vi "Launcher - Main View.vi"() -> ()   [LabVIEW 2018]
uses:
  <vilib>/Utility/miscctls.llb/LVPointTypeDef.ctl
  Workers/Main View/Main View.lvclass
  D:/Program Files (x86)/National Instruments/LabVIEW 2018/vi.lib/addons/_Workers/Library/Classes/Worker/Worker.lvclass
  Workers/Aging View/Aging View.lvclass
  Workers/Query Data/Query Data.lvclass
  Workers/Save Data/Save Data.lvclass
  Workers/Acquire Data/Acquire Data.lvclass
  Workers/About View/About View.lvclass
  Workers/Settings View/Settings View.lvclass
  <vilib>/addons/_Workers/Library/Classes/Message/Enqueue Message to Self v2.vi
  <vilib>/addons/_Workers/Library/Classes/Message/Message.lvclass
  <vilib>/addons/_Workers/Debugger/Debug Client/Debug Client.lvlib
  D:/Program Files (x86)/National Instruments/LabVIEW 2018/vi.lib/addons/_Workers/Library/Classes/Workers Object/Workers Object.lvclass
panel:
  out "About View":picture caption="[About]"
  out "Query View":picture caption="[Query]"
  out "Settings View":picture caption="[Settings]"
  out "Aging View":picture caption="[Aging]"
  out "error out":errorcluster
  # "Workers Demo - Aging Test"
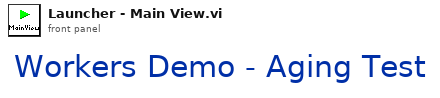
[diagram p1: front panel]
types:
  T1 = enum32{"Invalid", "Standard", "Closed", "Hidden", "Minimized", "Maximized"}
  T2 = typedef "LVPointTypeDef.ctl" = cluster{"Horizontal":i16, "Vertical":i16}
  T3 = typedef "Workers.lvlib/Case Label.ctl" = string
  T4 = typedef "imagedata.ctl" = cluster{"image type":i32, "image depth":i32, "image":u8[], "mask":u8[], "colors":u32[], "Rectangle":cluster{"left":i16, "top":i16, "right":i16, "bottom":i16}}
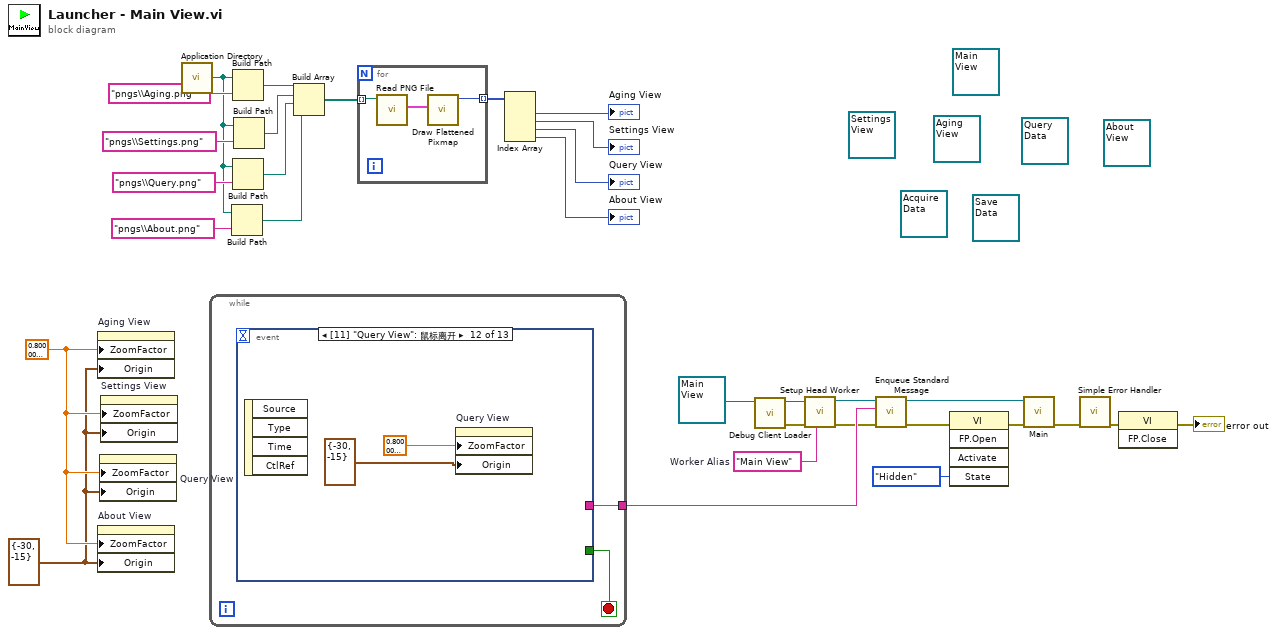
[diagram p0: block diagram]
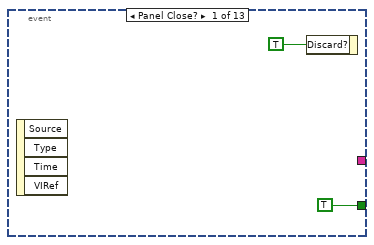
[diagram p2: hidden frame]
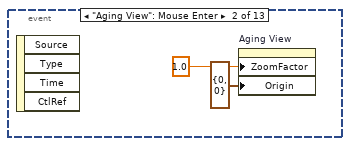
[diagram p3: hidden frame]
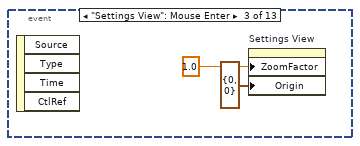
[diagram p4: hidden frame]
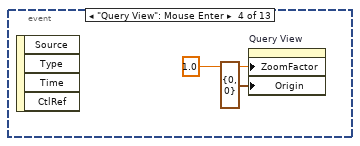
[diagram p5: hidden frame]
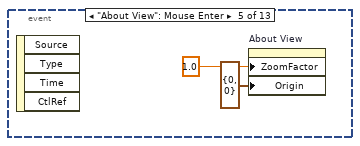
[diagram p6: hidden frame]
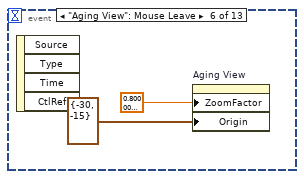
[diagram p7: hidden frame]
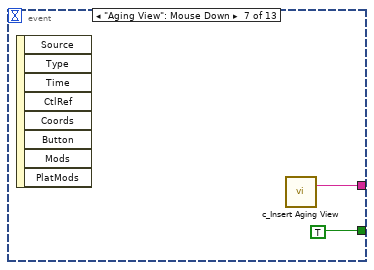
[diagram p8: hidden frame]
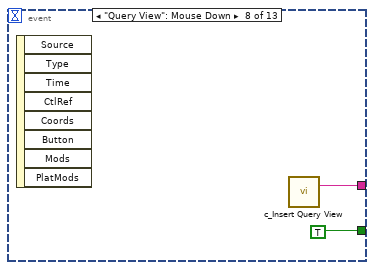
[diagram p9: hidden frame]
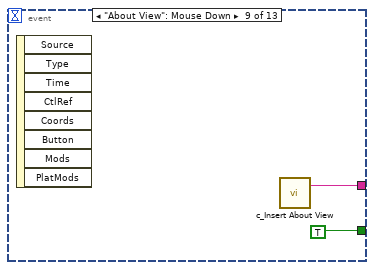
[diagram p10: hidden frame]
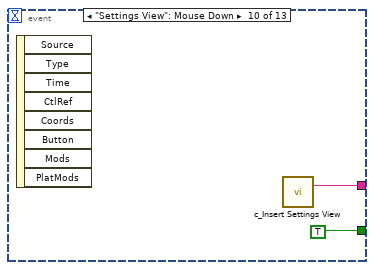
[diagram p11: hidden frame]
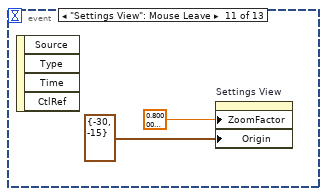
[diagram p12: hidden frame]
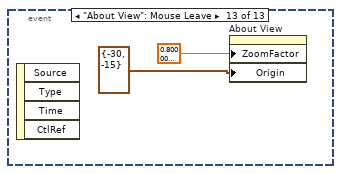
[diagram p13: hidden frame]
diagram:
  (unwired) refnum<class "Settings View.lvclass"> refnum ("Settings View.lvclass")
  (unwired) refnum<class "About View.lvclass"> refnum ("About View.lvclass")
  (unwired) refnum<class "Acquire Data.lvclass"> refnum ("Acquire Data.lvclass")
  (unwired) refnum<class "Save Data.lvclass"> refnum ("Save Data.lvclass")
  (unwired) refnum<class "Query Data.lvclass"> refnum ("Query Data.lvclass")
  (unwired) refnum<class "Main View.lvclass"> refnum ("Main View.lvclass")
  (unwired) refnum<class "Aging View.lvclass"> refnum ("Aging View.lvclass")
  w13 = "Main View"  # Worker Alias
  w15 = T2 {"Horizontal"=-30, "Vertical"=-15} ("Origin")
  w21 = sgl 0.8 ("Zoom Factor")
  n1 = property on="Aging View" class="Pict"("ZoomFactor"=w21, "Origin"=w15) -> ()  [unwired: 2 in, 2 out]
  n2 = property on="About View" class="Pict"("ZoomFactor"=w21, "Origin"=w15) -> ()  [unwired: 2 in, 2 out]
  n3 = property on="Query View" class="Pict"("ZoomFactor"=w21, "Origin"=w15) -> ()  [unwired: 2 in, 2 out]
  n4 = property on="Settings View" class="Pict"("ZoomFactor"=w21, "Origin"=w15) -> ()  [unwired: 2 in, 2 out]
  n5 = call <vilib>:"Application Directory.vi"() -> ("Application Directory"=w27:path)
  n6 = while {
    tunnel: [w32] -> w6
    stop <- w33 stop-if-true
    n7 = event shown="[11] \"Query View\": 鼠标离开" {
      selector: _ -> [_ _ _ _ _ _ _ _ _ _ _ _ _]
      dyn-events: _ -> [_ _ _ _ _ _ _ _ _ _ _ _ _]
      timeout: _ -> [_ _ _ _ _ _ _ _ _ _ _ _ _]
      tunnel: [TRUE _ _ _ _ _ TRUE TRUE TRUE TRUE _ _ _] -> w33
      tunnel: [_ _ _ _ _ _ w46 w48 w50 w52 _ _ _] -> w32
      event Panel Close? {
        n8 = event-data() -> ()  [unwired: 1 in, 4 out]
        n9 = event-data("Discard?"=TRUE) -> ()  [unwired: 1 in, 1 out]
      }
      event "Aging View": Mouse Enter {
        n10 = event-data() -> ()  [unwired: 1 in, 4 out]
        n11 = property on="Aging View" class="Pict"("ZoomFactor"=sgl 1.0 ("Zoom Factor"), "Origin"=T2 {"Horizontal"=0, "Vertical"=0}) -> ()  [unwired: 2 in, 2 out]
      }
      event "Settings View": Mouse Enter {
        n12 = event-data() -> ()  [unwired: 1 in, 4 out]
        n13 = property on="Settings View" class="Pict"("ZoomFactor"=sgl 1.0 ("Zoom Factor"), "Origin"=T2 {"Horizontal"=0, "Vertical"=0}) -> ()  [unwired: 2 in, 2 out]
      }
      event "Query View": Mouse Enter {
        n14 = event-data() -> ()  [unwired: 1 in, 4 out]
        n15 = property on="Query View" class="Pict"("ZoomFactor"=sgl 1.0 ("Zoom Factor"), "Origin"=T2 {"Horizontal"=0, "Vertical"=0}) -> ()  [unwired: 2 in, 2 out]
      }
      event "About View": Mouse Enter {
        n16 = event-data() -> ()  [unwired: 1 in, 4 out]
        n17 = property on="About View" class="Pict"("ZoomFactor"=sgl 1.0 ("Zoom Factor"), "Origin"=T2 {"Horizontal"=0, "Vertical"=0}) -> ()  [unwired: 2 in, 2 out]
      }
      event "Aging View": Mouse Leave {
        n18 = event-data() -> ()  [unwired: 1 in, 4 out]
        n19 = property on="Aging View" class="Pict"("ZoomFactor"=sgl 0.8 ("Zoom Factor"), "Origin"=T2 {"Horizontal"=-30, "Vertical"=-15}) -> ()  [unwired: 2 in, 2 out]
      }
      event "Aging View": Mouse Down {
        n20 = event-data() -> ()  [unwired: 1 in, 8 out]
        n21 = call "c_Insert Aging View.vi"() -> ("Case Label"=w46:T3)  [unwired: 1 in]
      }
      event "Query View": Mouse Down {
        n22 = event-data() -> ()  [unwired: 1 in, 8 out]
        n23 = call "c_Insert Query View.vi"() -> ("Case Label"=w48:T3)  [unwired: 1 in]
      }
      event "About View": Mouse Down {
        n24 = event-data() -> ()  [unwired: 1 in, 8 out]
        n25 = call "c_Insert About View.vi"() -> ("Case Label"=w50:T3)  [unwired: 1 in]
      }
      event "Settings View": Mouse Down {
        n26 = event-data() -> ()  [unwired: 1 in, 8 out]
        n27 = call "c_Insert Settings View.vi"() -> ("Case Label"=w52:T3)  [unwired: 1 in]
      }
      event "Settings View": Mouse Leave {
        n28 = event-data() -> ()  [unwired: 1 in, 4 out]
        n29 = property on="Settings View" class="Pict"("ZoomFactor"=sgl 0.8 ("Zoom Factor"), "Origin"=T2 {"Horizontal"=-30, "Vertical"=-15}) -> ()  [unwired: 2 in, 2 out]
      }
      event "Query View": Mouse Leave {
        n30 = event-data() -> ()  [unwired: 1 in, 4 out]
        n31 = property on="Query View" class="Pict"("ZoomFactor"=sgl 0.8 ("Zoom Factor"), "Origin"=T2 {"Horizontal"=-30, "Vertical"=-15}) -> ()  [unwired: 2 in, 2 out]
      }
      event "About View": Mouse Leave {
        n32 = event-data() -> ()  [unwired: 1 in, 4 out]
        n33 = property on="About View" class="Pict"("ZoomFactor"=sgl 0.8 ("Zoom Factor"), "Origin"=T2 {"Horizontal"=-30, "Vertical"=-15}) -> ()  [unwired: 2 in, 2 out]
      }
    }
  }
  n34 = Build Path(base path=w27, name or relative path="pngs\\About.png") -> (appended path=w23:path)
  n35 = Build Path(base path=w27, name or relative path="pngs\\Aging.png") -> (appended path=w26:path)
  n36 = Build Path(base path=w27, name or relative path="pngs\\Query.png") -> (appended path=w24:path)
  n37 = Build Path(base path=w27, name or relative path="pngs\\Settings.png") -> (appended path=w25:path)
  n38 = Build Array(w26, w25, w24, w23) -> (w22:path[])
  n39 = for {
    tunnel: w22 -> [w62] mode=indexing
    tunnel: [w60] -> w20 mode=indexing
    n40 = call <vilib>:"Read PNG File.vi"("path to PNG file"=w62) -> ("image data"=w61:T4)  [unwired: 8 in, 2 out]
    n41 = call <vilib>:"Draw Flattened Pixmap.vi"("image data"=w61) -> ("new picture"=w60:picture)  [unwired: 8 in]
  }
  n42 = Index Array(array=w20) -> (element #1=→"Aging View":picture, element #2=→"Settings View":picture, element #3=→"Query View":picture, element #4=→"About View":picture)  [unwired: 4 in]
  n43 = call <vilib>:"Debug Client Loader.vi"("Worker"=refnum<class "Main View.lvclass"> refnum ("Worker User Object")) -> ("error out"=w3:errorcluster, "Worker out"=w1:refnum<class "Main View.lvclass">)  [unwired: 9 in]
  n44 = call-dynamic "Setup Head Worker.vi"("Worker Alias"=w13, "error in"=w3, "Worker"=w1) -> ("error out"=w5:errorcluster, "Worker out"=w8:refnum<class "Main View.lvclass">)  [unwired: 7 in]
  n45 = call-poly <vilib>:"Enqueue Standard Message.vi"("Worker"=w8, "error in"=w5, "Case Label"=w6) -> ("error out"=w4:errorcluster, "dup Worker out"=w7:refnum<class "Main View.lvclass">)  [unwired: 7 in]
  n46 = invoke class="VI" method="FP.Open"(error in=w4, "State"=T1."Hidden") -> (error out=w12:errorcluster)  [unwired: 3 in, 4 out]
  n47 = call-dynamic "Main.vi"("error in"=w12, "Main View in"=w7) -> ("error out"=w14:errorcluster)  [unwired: 8 in, 1 out]
  n48 = call <vilib>:"Simple Error Handler.vi"("error in (no error)"=w14) -> ("error out"=w10:errorcluster)  [unwired: 4 in, 4 out]
  n49 = invoke class="VI" method="FP.Close"(error in=w10) -> (error out=→"error out":errorcluster)  [unwired: 2 in, 2 out]
